vi "FeedForward.vi"(10 "backward?":bool, 11 "Current Time":dbl) -> (3 "f(t)":sgl)   [LabVIEW 2016]
uses:
  <vilib>/NXT/Dual Mode Library/prims/inRangeAndCoerce/inRangeAndCoerce_float.vi
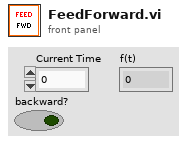
[diagram p1: front panel]
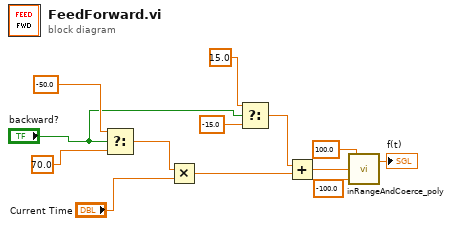
[diagram p0: block diagram]
diagram:
  n1 = Select(t=-50.0 ("Drive"), s="backward?", f=70.0 ("Drive")) -> (s? t:f=w7:dbl)
  n2 = Multiply(x=w7, y="Current Time") -> (x*y=w5:dbl)
  n3 = Select(t=15.0 ("x"), s="backward?", f=-15.0) -> (s? t:f=w1:dbl)
  n4 = Add(x=w1, y=w5) -> (x+y=w6:dbl)
  n5 = call-poly <vilib>:"inRangeAndCoerce_poly.vi"("lower limit"=sgl -100.0, "x"=w6, "upper limit"=sgl 100.0) -> ("coerced(x)"=→"f(t)":sgl)  [unwired: 1 out]
